vi "Close stdin.vi"(8 "error in (no error)":errorcluster, 11 "subprocess in":refnum<class "Subprocess.lvclass">) -> (0 "error out":errorcluster, 3 "subprocess out":refnum<class "Subprocess.lvclass">)   [LabVIEW 2020, in "NI_Subprocess.lvlib" / "Subprocess.lvclass"]
doc: "Flush buffers to the subprocess's stdin, then closes it."
uses:
  <vilib>/Subprocess/Subprocess/Subprocess.lvclass
  <vilib>/Subprocess/Subprocess/Subprocess.lvclass/Subprocess.ctl
  lviosrg.dll
  <vilib>/Utility/error.llb/Error Cluster From Error Code.vi
  <vilib>/ErrorRing/Error Ring.xnode
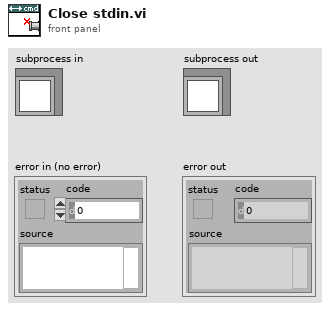
[diagram p1: front panel]
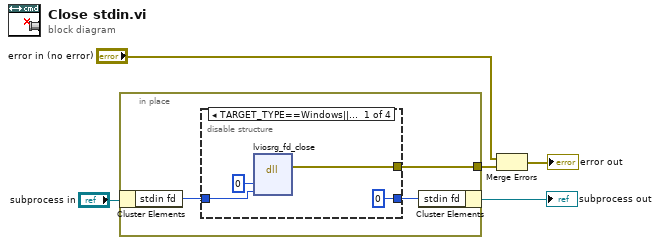
[diagram p0: block diagram]
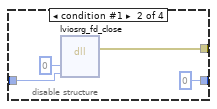
[diagram p2: hidden frame]
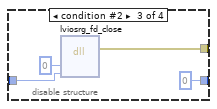
[diagram p3: hidden frame]
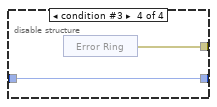
[diagram p4: hidden frame]
diagram:
  n1 = in-place {
    in-place-border: [w6] -> w4
    n2 = in-place-cluster #1("subprocess in") -> ("stdin fd"=w8:u64)
    n3 = disable-structure shown="TARGET_TYPE==Windows||OS==Win" {
      disable-tunnel: w8 -> [w11 w15 w19 w22]
      disable-tunnel: [0 ("stdin fd") 0 ("stdin fd") 0 ("stdin fd") w22] -> w7
      disable-tunnel: [w9 w13 w17 w21] -> w6
      frame condition #0 (active) {
        n4 = dll-call lib="lviosrg.*" fn="lviosrg_fd_close"("errno"=0, "fd"=w11) -> (error out=w9:errorcluster)  [unwired: 6 in, 1 out]
      }
      frame condition #1 {
        n5 = dll-call lib="lviosrg.*" fn="lviosrg_fd_close"("errno"=0, "fd"=w15) -> (error out=w13:errorcluster)  [unwired: 6 in, 1 out]
      }
      frame condition #2 {
        n6 = dll-call lib="lviosrg.*" fn="lviosrg_fd_close"("errno"=0, "fd"=w19) -> (error out=w17:errorcluster)  [unwired: 6 in, 1 out]
      }
      frame condition #3 {
        n7 = xnode "Error Ring"() -> ("error out"=w21:errorcluster)
      }
    }
    n8 = in-place-cluster #1("stdin fd"=w7) -> (→"subprocess out":refnum<class "Subprocess.lvclass">)
  }
  n9 = Merge Errors("error in (no error)", w4) -> (→"error out":errorcluster)
